vi "SR630GPIB.vi"() -> ()   [LabVIEW 2012]
doc: "This example requires NI-488.2 and NI-VISA to be installed on the system. The example shows how to communicate with a GPIB instrument using VISA reads, writes, and formatting functions on the returned data. This example will work using an NI Instrument Simulator or other instrument that has similar behavior."
panel:
  out "Read Buffer":string
  in  "Write Buffer":string="SENS:DATA?"
  in  "VISA GPIB Resource":refnum<visa-resource-name>="GPIB0::2::INSTR"
  # "On Windows/Linux, consider using the Instrument Driver Finder (Help>>Find Instrument Drivers) to search for an instrument driver for your instrument."
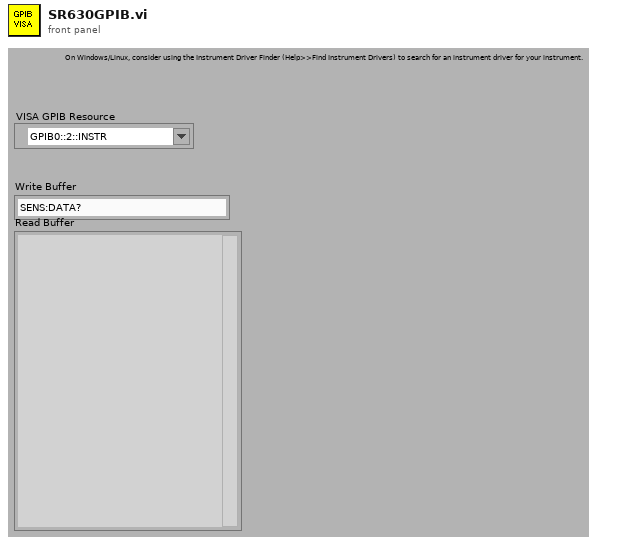
[diagram p1: front panel]
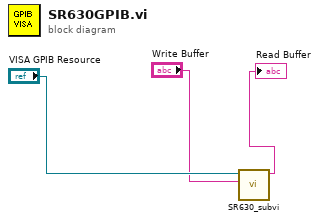
[diagram p0: block diagram]
diagram:
  n1 = call "SR630_subvi.vi"("Write Buffer"="Write Buffer", "VISA Refnum in"="VISA GPIB Resource") -> ("read buffer"=→"Read Buffer":string)  [unwired: 9 in]
